vi "SaveConfig.vi"(8 "error in (no error)":errorcluster, 11 "GRMActor in":refnum<class "MicroscopeController.lvclass">) -> (0 "error out":errorcluster, 3 "GRMActor out":refnum<class "MicroscopeController.lvclass">)   [LabVIEW 2020, in "MicroscopeController.lvlib" / "MicroscopeController.lvclass"]
uses:
  MicroscopeController.lvclass
  MicroscopeController.lvclass/MicroscopeController.ctl
  Model/Hardware Abstraction Layer/Component/GenericActor/GenericActor/GenericController.lvclass
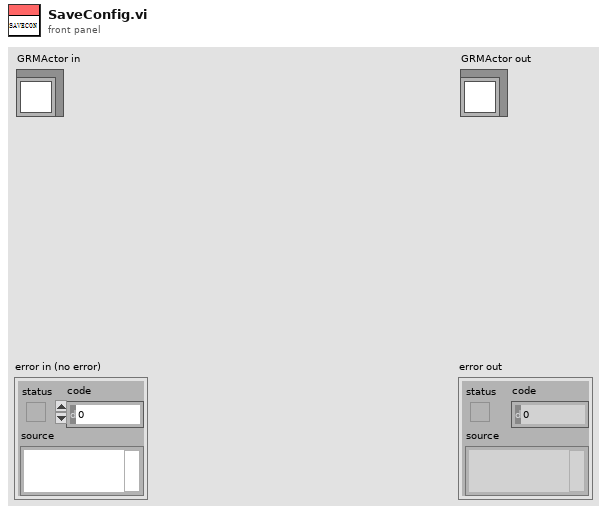
[diagram p1: front panel]
types:
  T1 = typedef "NI_LVConfig.lvlib/Config Data RefNum.ctl" = refnum<k1>
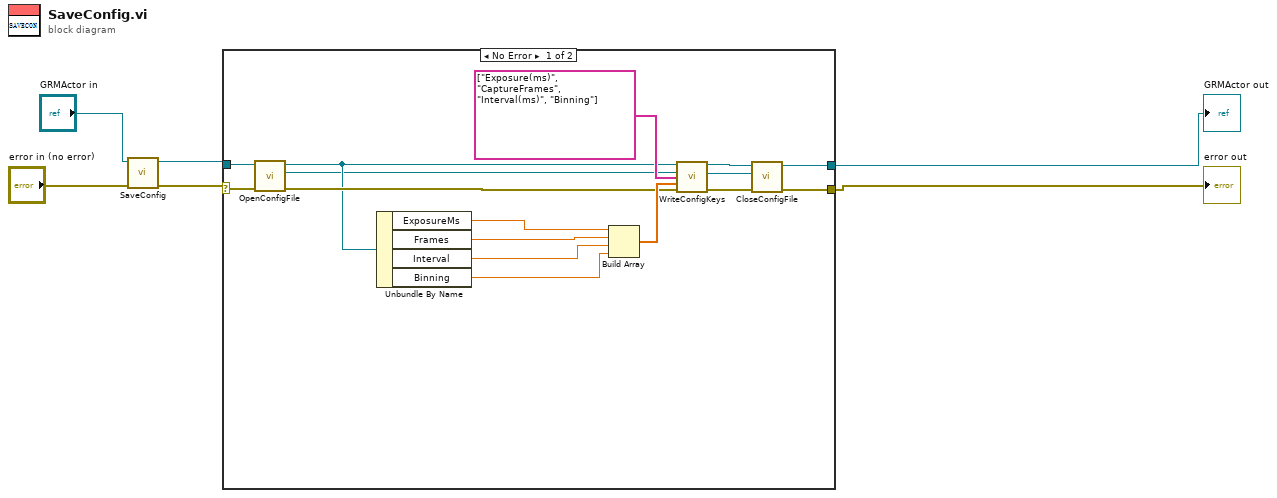
[diagram p0: block diagram]
diagram:
  n1 = call-parent "SaveConfig.vi"("error in (no error)"="error in (no error)", "GRMActor in"="GRMActor in") -> ("error out"=w3:errorcluster, "GRMActor out"=w4:refnum<class "MicroscopeController.lvclass">)  [unwired: 8 in]
  n2 = case shown="No Error" w3 {
    selector: w3 -> [w22 w23]
    tunnel: [w14 w23] -> w1
    tunnel: [w12 w24] -> w2
    tunnel: w4 -> [w11 w24]
    frame No Error {
      n3 = call-dynamic "OpenConfigFile.vi"("error in (no error)"=w22, "GRMActor in"=w11) -> ("error out"=w15:errorcluster, "refnum"=w9:T1, "GRMActor out"=w10:refnum<class "MicroscopeController.lvclass">)  [unwired: 7 in]
      n4 = Unbundle By Name(w10) -> ("ExposureMs"=w19:dbl, "Frames"=w18:dbl, "Interval"=w17:dbl, "Binning"=w7:dbl)
      n5 = Build Array(w19, w18, w17, w7) -> (w16:dbl[])
      n6 = call-dynamic "WriteConfigKeys.vi"("GRMActor in"=w10, "Config Refnum"=w9, "Keys"=string[] ["Exposure(ms)", "CaptureFrames", "Interval(ms)", "Binning"], "IntValue"=w16, "error in (no error)"=w15) -> ("GRMActor out"=w13:refnum<class "MicroscopeController.lvclass">, "Config Refnum dup"=w8:T1, "error out"=w21:errorcluster)  [unwired: 8 in]
      n7 = call-dynamic "CloseConfigFile.vi"("error in (no error)"=w21, "refnum"=w8, "GRMActor in"=w13) -> ("error out"=w14:errorcluster, "GRMActor out"=w12:refnum<class "MicroscopeController.lvclass">)  [unwired: 7 in]
    }
    frame Error {
    }
  }
  "error out" <- w1
  "GRMActor out" <- w2
